vi "NonDuplicateArrays.vi"(8 "error in":errorcluster, 9 "string in":string, 11 "array in":string[](array[string])) -> (0 "error out":errorcluster, 3 "array out":string[](array[string]))   [LabVIEW 2013, in "NISE_CEF_TreeControl.lvlib"]
doc: "This Vi checks if the string exist in the array, if it doesnt it adds it to the array."
uses:
  NISE_CEF_TreeControl.lvlib
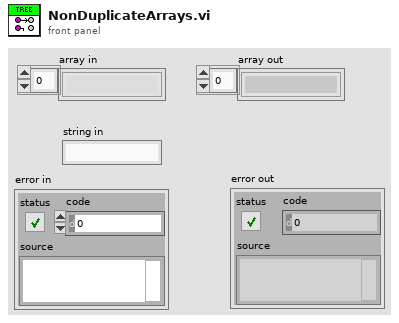
[diagram p1: front panel]
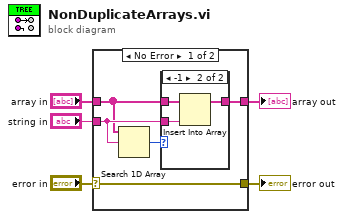
[diagram p0: block diagram]
diagram:
  n1 = case shown="No Error" "error in" {
    selector: "error in" -> [w7 w16]
    tunnel: "string in" -> [w10 _]
    tunnel: "array in" -> [w9 w15]
    tunnel: [w7 w16] -> w2
    tunnel: [w6 w15] -> w1
    frame No Error {
      n2 = Search 1D Array(1D array=w9, element=w10) -> (index of element=w8:i32)  [unwired: 1 in]
      n3 = case shown="-1" w8 {
        tunnel: [w11 w13] -> w6
        tunnel: w9 -> [w11 w14]
        tunnel: w10 -> [_ w12]
        frame 0, Default {
        }
        frame -1 {
          n4 = Insert Into Array(array=w14, new element=w12) -> (w13:string[])  [unwired: 1 in]
        }
      }
    }
    frame Error {
    }
  }
  "error out" <- w2
  "array out" <- w1
